vi "NiFPGA Read.vi"   [LabVIEW 2010, in "FPGA Interface Wrapper.lvlib"]
doc: "Reads data from an indicator"
uses:
  <userlib>/_FPGA Interface Advanced Tools/FPGA Interface Wrapper/FPGA Interface Wrapper.lvlib
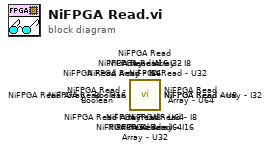
[diagram p0: block diagram]
diagram:
  n1 = call <userlib>:"NiFPGA Read - U64.vi"() -> ()  [unwired: 9 in, 3 out]
  n2 = call <userlib>:"NiFPGA Read - U32.vi"() -> ()  [unwired: 9 in, 3 out]
  n3 = call <userlib>:"NiFPGA Read - U16.vi"() -> ()  [unwired: 9 in, 3 out]
  n4 = call <userlib>:"NiFPGA Read - U8.vi"() -> ()  [unwired: 9 in, 3 out]
  n5 = call <userlib>:"NiFPGA Read - I64.vi"() -> ()  [unwired: 9 in, 3 out]
  n6 = call <userlib>:"NiFPGA Read - I32.vi"() -> ()  [unwired: 9 in, 3 out]
  n7 = call <userlib>:"NiFPGA Read - I16.vi"() -> ()  [unwired: 9 in, 3 out]
  n8 = call <userlib>:"NiFPGA Read - I8.vi"() -> ()  [unwired: 9 in, 3 out]
  n9 = call <userlib>:"NiFPGA Read - Boolean.vi"() -> ()  [unwired: 9 in, 3 out]
  n10 = call <userlib>:"NiFPGA Read Array - U64.vi"() -> ()  [unwired: 9 in, 3 out]
  n11 = call <userlib>:"NiFPGA Read Array - U32.vi"() -> ()  [unwired: 9 in, 3 out]
  n12 = call <userlib>:"NiFPGA Read Array - U16.vi"() -> ()  [unwired: 9 in, 3 out]
  n13 = call <userlib>:"NiFPGA Read Array - U8.vi"() -> ()  [unwired: 9 in, 3 out]
  n14 = call <userlib>:"NiFPGA Read Array - I64.vi"() -> ()  [unwired: 9 in, 3 out]
  n15 = call <userlib>:"NiFPGA Read Array - I32.vi"() -> ()  [unwired: 9 in, 3 out]
  n16 = call <userlib>:"NiFPGA Read Array - I16.vi"() -> ()  [unwired: 9 in, 3 out]
  n17 = call <userlib>:"NiFPGA Read Array - I8.vi"() -> ()  [unwired: 9 in, 3 out]
  n18 = call <userlib>:"NiFPGA Read Array - Boolean.vi"() -> ()  [unwired: 9 in, 3 out]
